vi "CombineSelectedShotandAllAcq.vi"(9 "Selected Shot Array":dbl[][](array[numeric]), 11 "AllAcq Array":dbl[][](array[numeric])) -> (2 "Combined Array":dbl[][](array[numeric]))   [LabVIEW 2020]
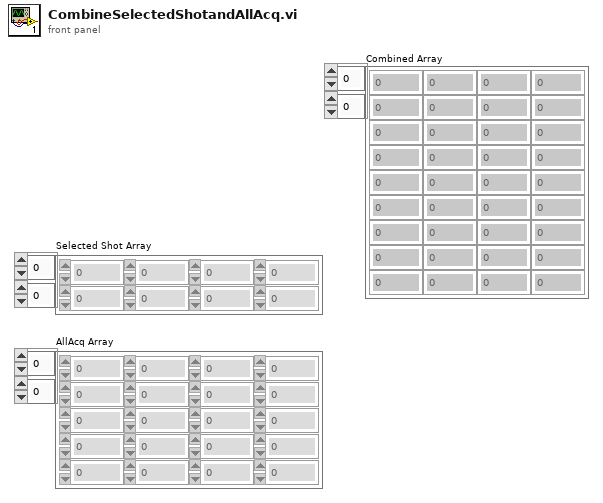
[diagram p1: front panel]
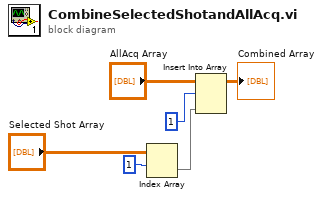
[diagram p0: block diagram]
diagram:
  n1 = Index Array(array="Selected Shot Array", index (row)=1) -> (element=w1:dbl[])  [unwired: 1 in]
  n2 = Insert Into Array(array="AllAcq Array", index (row)=1, new element=w1) -> (→"Combined Array":dbl[][])  [unwired: 1 in]
